vi "ReadWorkData.vi"(8 "error in (no error)":errorcluster, 11 "AbstractStep in":refnum<class "AbstractStep.lvclass">) -> (0 "error out":errorcluster, 2 "StepData.lvclass":refnum<class "StepData.lvclass">, 3 "AbstractStep out":refnum<class "AbstractStep.lvclass">)   [LabVIEW 2014, in "AbstractStep.lvclass"]
uses:
  AbstractStep.lvclass
  StepData/StepData.lvclass
  AbstractStep.lvclass/AbstractStep.ctl
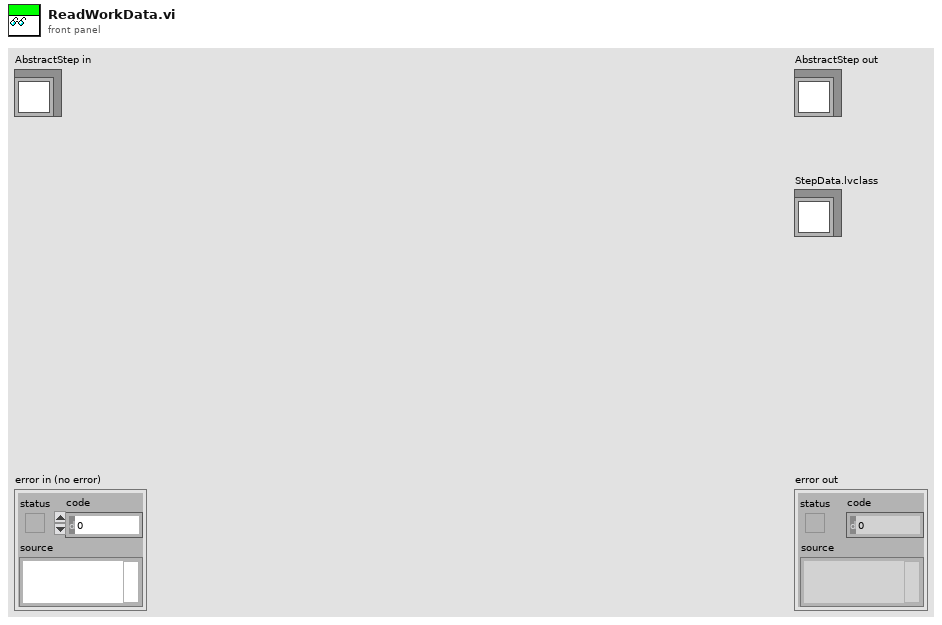
[diagram p1: front panel]
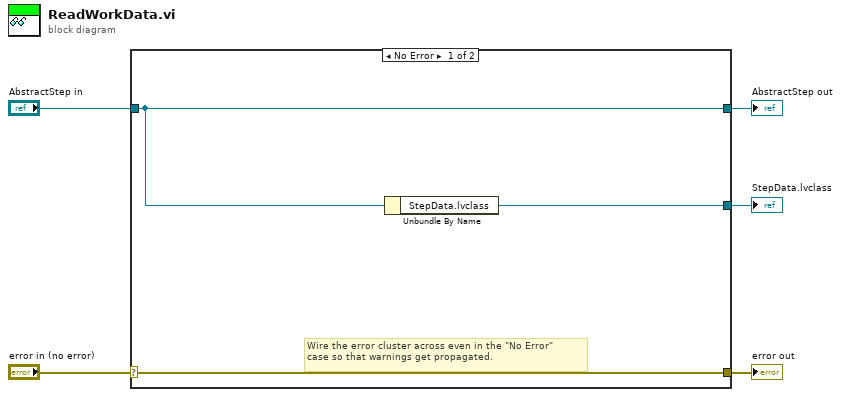
[diagram p0: block diagram]
diagram:
  n1 = case shown="No Error" "error in (no error)" {
    selector: "error in (no error)" -> [w8 w10]
    tunnel: [w8 w10] -> w4
    tunnel: [w7 w9] -> w2
    tunnel: "AbstractStep in" -> [w7 w9]
    tunnel: [w6 _] -> w1
    frame No Error {
      # "Wire the error cluster across even in the \"No Error\"\ncase so that warnings get propagated."
      n2 = Unbundle By Name(w7) -> ("StepData.lvclass"=w6:refnum<class "StepData.lvclass">)
    }
    frame Error {
    }
  }
  "error out" <- w4
  "AbstractStep out" <- w2
  "StepData.lvclass" <- w1
